vi "Integral.vi"() -> ()   [LabVIEW 2014]
uses:
  <vilib>/Analysis/8numeric.llb/1D Numeric Integration.vi
  <vilib>/express/express arith-compare/Formula/XNode/ExpressFormulaBlockNode.xnode
  <vilib>/Analysis/NI_AALPro.lvlib
panel:
  out "XY Graph":cluster{dbl[], "Integral X":dbl[]}[](graph)
  out "x":dbl[](array[numeric])
  out "Integral definida":dbl
  out "Erro":dbl
  out "My integral":dbl
  in  "Number of iterations":i32
  out "Numeric integral":dbl format="%0.4f"
  in  "Max":i32
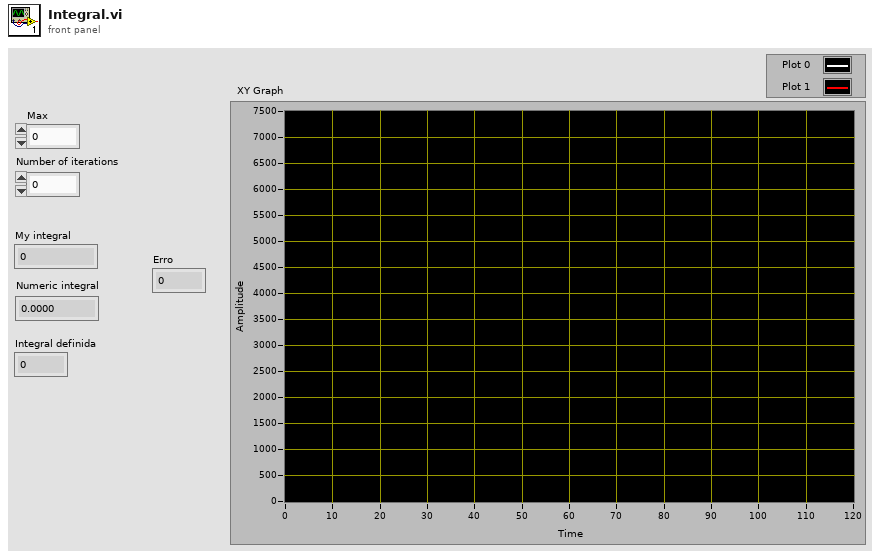
[diagram p1: front panel]
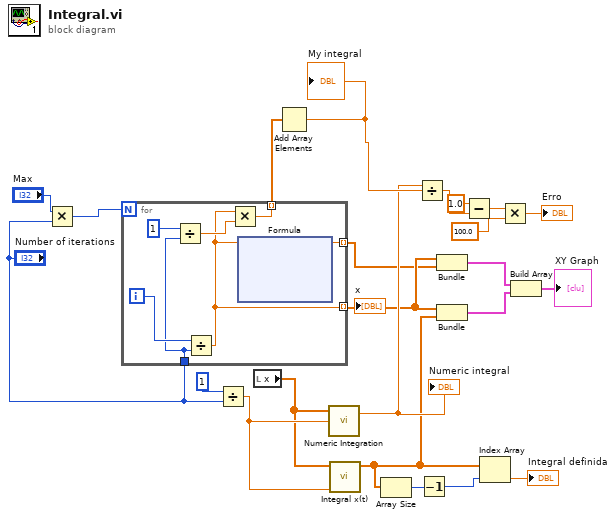
[diagram p0: block diagram]
diagram:
  n1 = Multiply(x="Max", y="Number of iterations") -> (x*y=w15:i32)
  n2 = for {
    N: w15 -> [_]
    tunnel: [w25] -> w6 mode=indexing
    tunnel: "Number of iterations" -> [w26]
    tunnel: [w29] -> w11 mode=indexing
    tunnel: [w24] -> w4 mode=indexing
    i -> [w30]
    n3 = Divide(x=1, y=w26) -> (x/y=w27:dbl)
    n4 = Divide(x=w30, y=w26) -> (x/y=w25:dbl)
    n5 = Multiply(x=w25, y=w27) -> (x*y=w29:dbl)
    n6 = xnode "Formula"("X1"=w25) -> ("Result"=w24:dbl)  [unwired: 1 in, 1 out]
  }
  "x" <- w6
  n7 = Divide(x=1, y="Number of iterations") -> (x/y=w10:dbl)
  n8 = local read "x"() -> (w7:dbl[])
  n9 = Add Array Elements(numeric array=w11) -> (sum=w17:dbl)
  "My integral" <- w17
  n10 = call-poly <vilib>:"Numeric Integration.vi"("dt"=w10, "Input Array"=w7) -> ("result"=w16:dbl)  [unwired: 1 in, 1 out]
  "Numeric integral" <- w16
  n11 = call <vilib>:"Integral x(t).vi"("dt"=w10, "X"=w7) -> ("Integral X"=w5:dbl[])  [unwired: 8 in, 1 out]
  n12 = Array Size(array=w5) -> (size(s)=w14:i32)
  n13 = Divide(x=w16, y=w17) -> (x/y=w21:dbl)
  n14 = Decrement(x=w14) -> (x-1=w13:i32)
  n15 = Bundle(w6, w4) -> (w3:cluster{dbl[], dbl[]})  [unwired: 1 in]
  n16 = Bundle(w6, "Integral X"=w5) -> (w2:cluster{dbl[], "Integral X":dbl[]})  [unwired: 1 in]
  n17 = Subtract(x=1.0 ("x/y"), y=w21) -> (x-y=w20:dbl)
  n18 = Index Array(array=w5, index=w13) -> (element=→"Integral definida":dbl)
  n19 = Multiply(x=w20, y=100.0) -> (x*y=→"Erro":dbl)
  n20 = Build Array(w3, w2) -> (→"XY Graph":cluster{dbl[], "Integral X":dbl[]}[])
